vi "calibratePhase.vi"(8 "error in (no error)":errorcluster, 10 "value":string, 11 "RfOutputChannel in":refnum<class "RfOutputChannel.lvclass">) -> (0 "error out":errorcluster, 2 "Phase":dbl, 3 "RfOutputChannel out":refnum<class "RfOutputChannel.lvclass">)   [LabVIEW 2009, in "Tools.lvlib" / "DatabaseHelpers.lvlib" / "RfOutputChannel.lvclass"]
uses:
  RfOutputChannel.lvclass
  RfOutputChannel.lvclass/RfOutputChannel.ctl
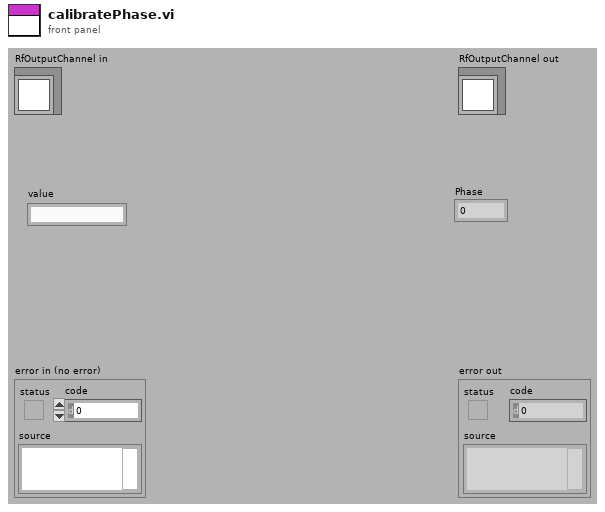
[diagram p1: front panel]
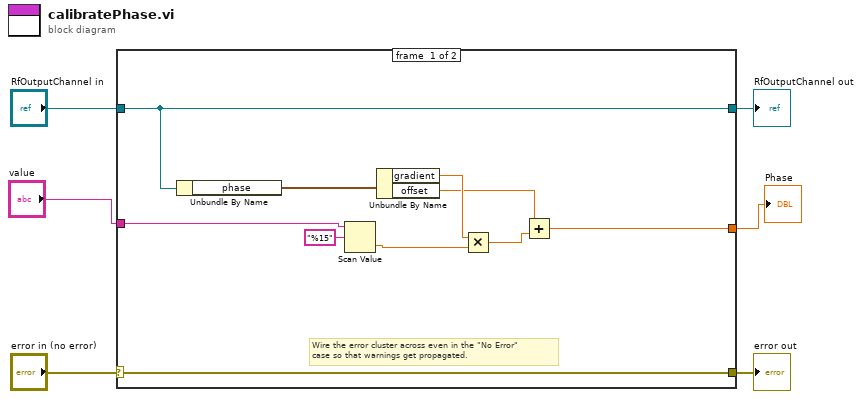
[diagram p0: block diagram]
diagram:
  n1 = case shown="No Error" "error in (no error)" {
    selector: "error in (no error)" -> [w16 w18]
    tunnel: [w16 w18] -> w5
    tunnel: [w9 w17] -> w3
    tunnel: "RfOutputChannel in" -> [w9 w17]
    tunnel: "value" -> [w8 _]
    tunnel: [w7 _] -> w1
    frame #0 {
      # "Wire the error cluster across even in the \"No Error\"\ncase so that warnings get propagated."
      n2 = Unbundle By Name(w9) -> ("phase"=w10:cluster{"gradient":dbl, "offset":dbl})
      n3 = Scan Value(string=w8, format string="%15") -> (value=w13:dbl)  [unwired: 1 in, 1 out]
      n4 = Unbundle By Name(w10) -> ("gradient"=w14:dbl, "offset"=w11:dbl)
      n5 = Multiply(x=w14, y=w13) -> (x*y=w12:dbl)
      n6 = Add(x=w11, y=w12) -> (x+y=w7:dbl)
    }
    frame #1 {
    }
  }
  "error out" <- w5
  "RfOutputChannel out" <- w3
  "Phase" <- w1
